vi "errori soglie calibrazioni.vi"(10 "millennio":i32=2000, 11 "PAGINE TRASDUTTORI":string[][](array[string])) -> (3 "Array errori":cluster{"tipo errore":i32, "index":i32}[](array[cluster]))   [LabVIEW 2019]
uses:
  <vilib>/Utility/miscctls.llb/LVDateTimeRec.ctl
panel:
  # "0 = calibrazione scaduta\n1 = scadenza entro 1 mese\n2 = calibrazione ok"
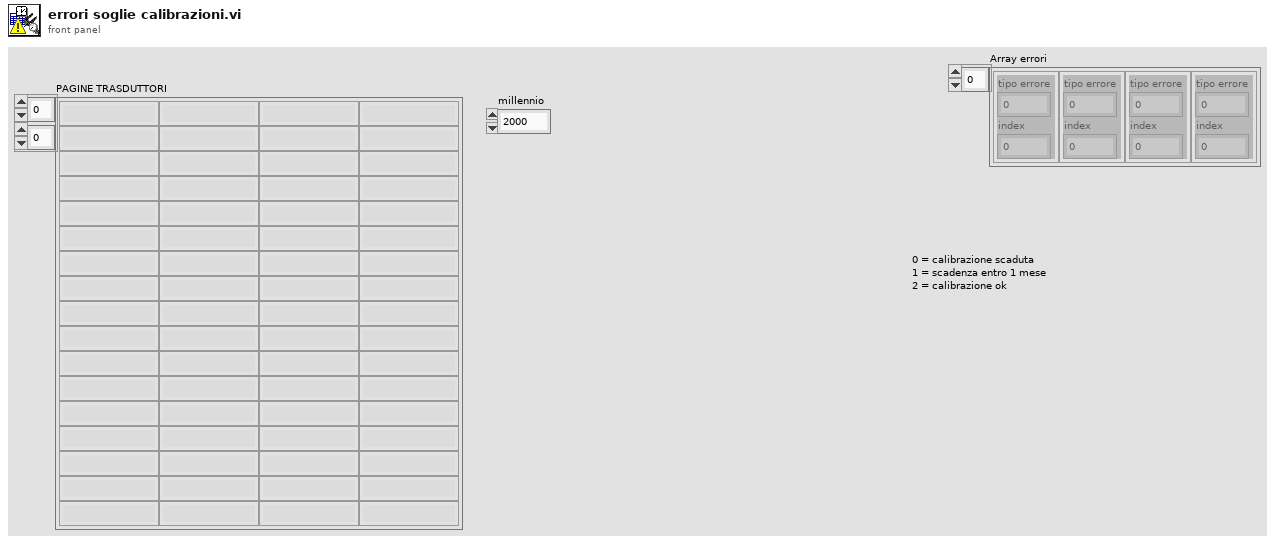
[diagram p1: front panel]
types:
  T1 = typedef "LVDateTimeRec.ctl" = cluster{"fractional second":dbl, "second":i32, "minute":i32, "hour":i32, "day of month":i32, "month":i32, "year":i32, "day of week":i32, "day of year":i32, "DST":i32}
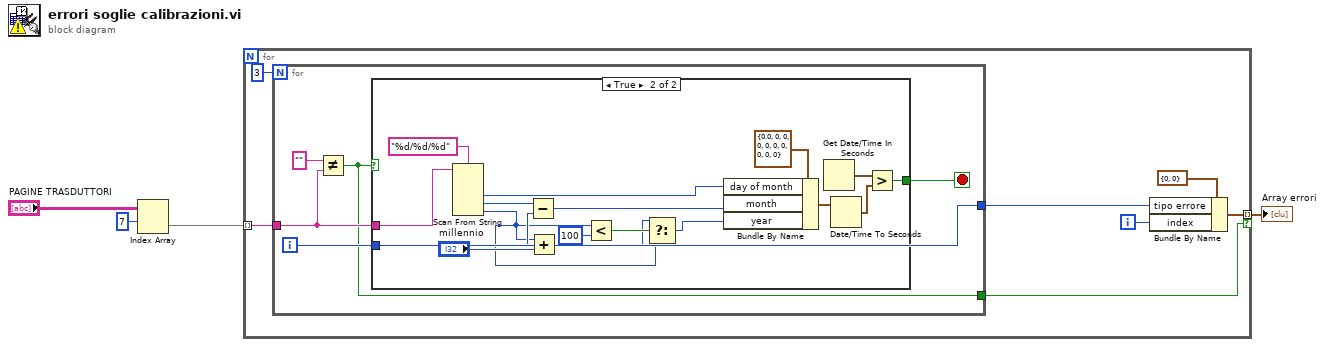
[diagram p0: block diagram]
diagram:
  n1 = Index Array(array="PAGINE TRASDUTTORI", index (row)=7) -> (element=w1:string[])  [unwired: 1 in]
  n2 = for {
    tunnel: w1 -> [w11] mode=indexing
    tunnel: [w6] -> w2 mode=indexing if=w5
    i -> [w7]
    n3 = for {
      N: 3 -> [_]
      tunnel: w11 -> [w14]
      tunnel: [w16] -> w8
      tunnel: [w12] -> w5
      i -> [w16]
      stop <- w15 stop-if-true
      n4 = Not Equal?(x="", y=w14) -> (x != y?=w12:bool)
      n5 = case shown="True" w12 {
        tunnel: w14 -> [_ w27]
        tunnel: w16 -> [_ w24]
        tunnel: [_ w23] -> w15
        frame False {
        }
        frame True {
          n6 = Scan From String(format string="%d/%d/%d", input string=w27) -> (output 1=w30:i32, output 2=w26:i32, output 3=w18:i32)  [unwired: 5 in, 3 out]
          n7 = Subtract(x=w26, y=w24) -> (x-y=w25:i32)
          n8 = Add(x=w18, y="millennio") -> (x+y=w19:i32)
          n9 = Less?(x=w18, y=100) -> (x < y?=w20:bool)
          n10 = Select(t=w19, s=w20, f=w18) -> (s? t:f=w17:i32)
          n11 = Bundle By Name(cluster=T1 {"fractional second"=0.0, "second"=0, "minute"=0, "hour"=0, "day of month"=0, "month"=0, "year"=0, "day of week"=0, "day of year"=0, "DST"=0} ("date time rec"), "day of month"=w30, "month"=w25, "year"=w17) -> (w31:T1)
          n12 = Get Date/Time In Seconds() -> (seconds since 1Jan1904=w32:timestamp)
          n13 = Date/Time To Seconds(2:w31) -> (0:w33:timestamp)  [unwired: 1 in]
          n14 = Greater?(x=w32, y=w33) -> (0:w23:bool)
        }
      }
    }
    n15 = Bundle By Name(cluster=cluster{"tipo errore":i32, "index":i32} {"tipo errore"=0, "index"=0}, "tipo errore"=w8, "index"=w7) -> (w6:cluster{"tipo errore":i32, "index":i32})
  }
  "Array errori" <- w2
